vi "Get All Tags in Memory.vi"(8 "error in (no error)":errorcluster, 11 "(Re)initialize?":bool) -> (0 "error out":errorcluster, 3 "CVT File Data":T1)   [LabVIEW 2020, in "Current Value Table(Rebuild).lvlib"]
doc: "This VI fetches all tags currently in the engine and generates a tag list similar to the function used to initialize the CVT. This is actually a functional global variable which stores all the tags and their indices. When the function is called the first time, or if the (re)initialize boolean is set, it will retrieve all tags from the CVT along with their indices. This process takes approximately 200 ms for 1000 tags on the cRIO 9076. Subsequent calls are much faster, as they simply read the required data from the CVT memblock."
uses:
  Current Value Table(Rebuild).lvlib
  Type Defs/Tag Grouping set.ctl
  Type Defs/Data Types.ctl
  Type Defs/File Format.ctl
  Type Defs/Single Tag.ctl
  FGVs/Tag Memory Methods.ctl
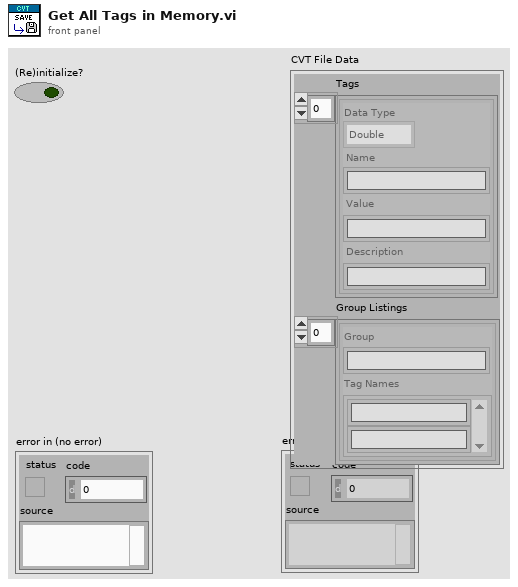
[diagram p1: front panel]
types:
  T1 = typedef "Current Value Table(Rebuild).lvlib/File Format.ctl" = cluster{"Tags":T2[], "Group Listings":T4[]}
  T2 = typedef "Current Value Table(Rebuild).lvlib/Single Tag.ctl" = cluster{"Data Type":T3, "Name":string, "Value":string, "Description":string}
  T3 = typedef "Current Value Table(Rebuild).lvlib/Data Types.ctl" = enum16{"Double", "Single", "I64", "I32", "I16", "I8", "U64", "U32", "U16", "U8", "String", "Boolean", "Array of U8", "Array of U16", "Array of U32", "Array of U64", "Array of I64", "Array of I32", "Array of I16", "Array of I8", "Array of Double", "Array of Single", "Array of Boolean", "Array of String"}
  T4 = typedef "Current Value Table(Rebuild).lvlib/Tag Grouping set.ctl" = cluster{"Group":string, "Tag Names":string[]}
  T5 = typedef "Current Value Table(Rebuild).lvlib/Tag in Memory.ctl" = cluster{"Index":i32, "Tag":T2}
  T6 = typedef "Current Value Table(Rebuild).lvlib/Tag Memory Methods.ctl" = enum16{"Clear", "Read Tag Index", "Read Tag Indices", "Generate Group", "Add Tag", "Overwrite Tag", "Read Description", "Get Stored Tags", "Write Description"}
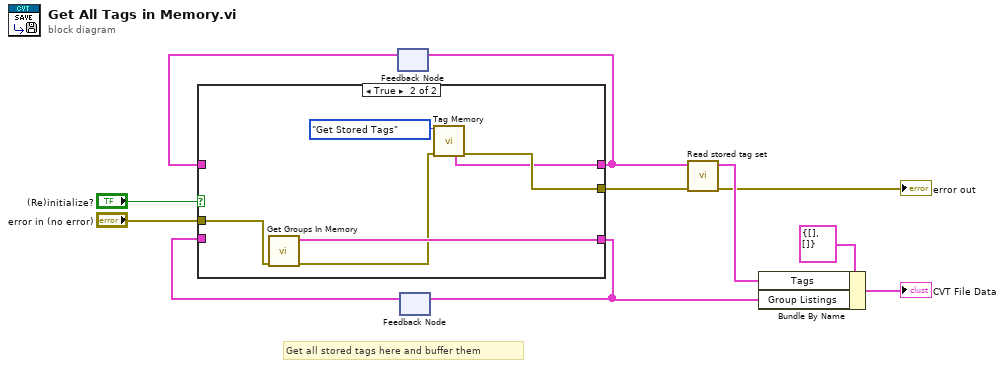
[diagram p0: block diagram]
diagram:
  # "Get all stored tags here and buffer them"
  n1 = feedback #1() -> (w9:T5[])  [unwired: 1 in]
  n2 = feedback #2() -> (w8:T4[])  [unwired: 1 in]
  n3 = case shown="True" "(Re)initialize?" {
    tunnel: "error in (no error)" -> [w14 w20]
    tunnel: [w14 w18] -> w2
    tunnel: [w13 w15] -> w4
    tunnel: w9 -> [w13 _]
    tunnel: [w12 w19] -> w6
    tunnel: w8 -> [w12 _]
    frame False {
    }
    frame True {
      n4 = call "Get Groups In Memory.vi"("error in (no error)"=w20) -> ("error out"=w16:errorcluster, "Groups In Memory"=w19:T4[])  [unwired: 9 in]
      n5 = call "Tag Memory.vi"("Method"=Tag_Memory_Methods."Get Stored Tags", "error in (no error)"=w16) -> ("Stored Tags"=w15:T5[], "error out"=w18:errorcluster)  [unwired: 8 in, 4 out]
    }
  }
  n6 = feedback-in #1(w4) -> ()
  n7 = feedback-in #2(w6) -> ()
  n8 = call "Read stored tag set.vi"("error in (no error)"=w2, "stored tags"=w4) -> ("error out"=→"error out":errorcluster, "Tags"=w3:T2[])  [unwired: 8 in]
  n9 = Bundle By Name(cluster=T1 {"Tags"=[], "Group Listings"=[]} ("File Format"), "Tags"=w3, "Group Listings"=w6) -> (→"CVT File Data":T1)
